vi "AnguloCupula.vi"(2 "ConstantesCupTel":T1={"QtdEtiq"=720, "EtiqMin"=1, "EtiqMax"=720, "Offset"=148.0, "SegurancaAjuste"=2.0, "LargTrapeira"=30.0, "ProjecaoTubo"=20.0, "RaioCupula"=7.525, "DistEntreEixos"=1.57, "AltBase"=0.3, "LATrad"=-0.3933}, 3 "AplicarAjuste":bool=TRUE, 4 "DEC":dbl, 5 "AH":dbl) -> (0 "PosCup":u16, 1 "AngCup":dbl)   [LabVIEW 2012]
panel:
  out "Aj_otimo":dbl
  # "(radianos)"
  # "(radianos)"
  # "(num. etiqueta)"
  # "(graus)"
  # "(graus)"
  # "Não"
  # "Sim"
  # "(graus)"
  # "(graus)"
  # "(metros)"
  # "(metros)"
  # "(metros)"
  # "(radianos)"
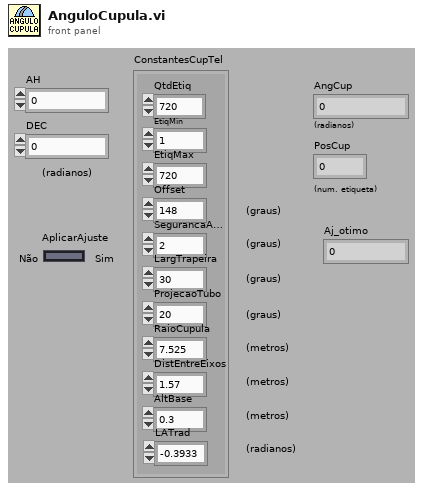
[diagram p1: front panel]
types:
  T1 = cluster{"QtdEtiq":u16, "EtiqMin":u16, "EtiqMax":u16, "Offset":dbl, "SegurancaAjuste":dbl, "LargTrapeira":dbl, "ProjecaoTubo":dbl, "RaioCupula":dbl, "DistEntreEixos":dbl, "AltBase":dbl, "LATrad":dbl}
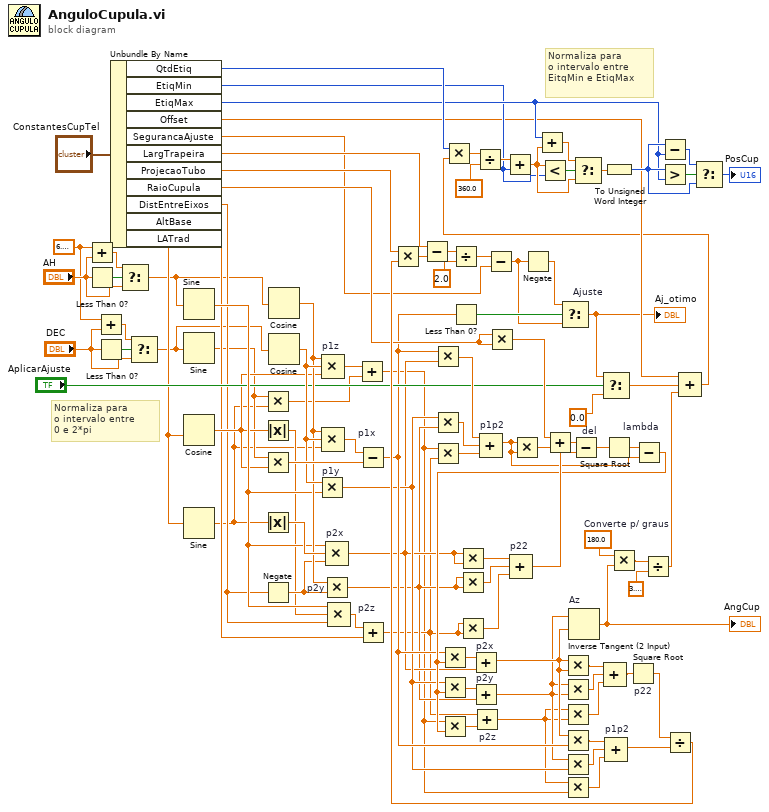
[diagram p0: block diagram]
diagram:
  w2 = 6.283185307179586
  w50 = 180.0  # Converte p/ graus
  # "Normaliza para\no intervalo entre\n0 e 2*pi"
  # "Normaliza para\no intervalo entre\nEitqMin e EtiqMax"
  n1 = Add(x=w2, y="AH") -> (x+y=w6:dbl)
  n2 = Less Than 0?(x="AH") -> (x < 0?=w9:bool)
  n3 = Add(x=w2, y="DEC") -> (x+y=w4:dbl)
  n4 = Less Than 0?(x="DEC") -> (x < 0?=w5:bool)
  n5 = Unbundle By Name("ConstantesCupTel") -> ("QtdEtiq"=w38:u16, "EtiqMin"=w30:u16, "EtiqMax"=w31:u16, "Offset"=w29:dbl, "SegurancaAjuste"=w28:dbl, "LargTrapeira"=w44:dbl, "ProjecaoTubo"=w43:dbl, "RaioCupula"=w42:dbl, "DistEntreEixos"=w41:dbl, "AltBase"=w40:dbl, "LATrad"=w39:dbl)
  n6 = Select(t=w6, s=w9, f="AH") -> (s? t:f=w8:dbl)
  n7 = Select(t=w4, s=w5, f="DEC") -> (s? t:f=w1:dbl)
  n8 = Sine(x=w8) -> (sin(x)=w93:dbl)
  n9 = Sine(x=w1) -> (sin(x)=w12:dbl)
  n10 = Cosine(x=w39) -> (cos(x)=w57:dbl)
  n11 = Sine(x=w39) -> (sin(x)=w11:dbl)
  n12 = Multiply(x=w12, y=w11) -> (x*y=w10:dbl)
  n13 = Absolute Value(x=w57) -> (abs(x)=w13:dbl)
  n14 = Multiply(x=w12, y=w57) -> (x*y=w99:dbl)
  n15 = Absolute Value(x=w11) -> (abs(x)=w95:dbl)
  n16 = Negate(x=w41) -> (-x=w91:dbl)
  n17 = Cosine(x=w8) -> (cos(x)=w94:dbl)
  n18 = Cosine(x=w1) -> (cos(x)=w97:dbl)
  n19 = Multiply "p1y"(x=w97, y=w93) -> (x*y=w25:dbl)
  n20 = Compound Arithmetic op=MULTIPLY "p1z"(w94, w97, w57) -> (w24:dbl)
  n21 = Compound Arithmetic op=MULTIPLY(w94, w97, w11) -> (w98:dbl)
  n22 = Multiply "p2y"(x=w94, y=w91) -> (x*y=w22:dbl)
  n23 = Compound Arithmetic op=MULTIPLY "p2x"(w93, w95, w91) -> (w23:dbl)
  n24 = Compound Arithmetic op=MULTIPLY(w93, w13, w41) -> (w96:dbl)
  n25 = Add(x=w24, y=w10) -> (x+y=w14:dbl)
  n26 = Subtract "p1x"(x=w98, y=w99) -> (x-y=w26:dbl)
  n27 = Add "p2z"(x=w96, y=w40) -> (x+y=w21:dbl)
  n28 = Multiply(x=w26, y=w23) -> (x*y=w86:dbl)
  n29 = Multiply(x=w25, y=w22) -> (x*y=w87:dbl)
  n30 = Multiply(x=w14, y=w21) -> (x*y=w92:dbl)
  n31 = Less Than 0?(x=w26) -> (x < 0?=w66:bool)
  n32 = Multiply(x=w23, y=w23) -> (x*y=w90:dbl)
  n33 = Multiply(x=w22, y=w22) -> (x*y=w89:dbl)
  n34 = Multiply(x=w21, y=w21) -> (x*y=w88:dbl)
  n35 = Compound Arithmetic op=ADD "p1p2"(w86, w87, w92) -> (w79:dbl)
  n36 = Multiply(x=w42, y=w42) -> (x*y=w83:dbl)
  n37 = Compound Arithmetic op=ADD "p22"(w90, w89, w88) -> (w82:dbl)
  n38 = Multiply(x=w79, y=w79) -> (x*y=w85:dbl)
  n39 = Add(x=w83, y=w85) -> (x+y=w84:dbl)
  n40 = Subtract "del"(x=w84, y=w82) -> (x-y=w81:dbl)
  n41 = Square Root(x=w81) -> (sqrt(x)=w80:dbl)
  n42 = Subtract "lambda"(x=w80, y=w79) -> (x-y=w60:dbl)
  n43 = Multiply(x=w26, y=w60) -> (x*y=w61:dbl)
  n44 = Multiply(x=w25, y=w60) -> (x*y=w78:dbl)
  n45 = Multiply(x=w14, y=w60) -> (x*y=w62:dbl)
  n46 = Add "p2x"(x=w61, y=w23) -> (x+y=w20:dbl)
  n47 = Add "p2y"(x=w78, y=w22) -> (x+y=w19:dbl)
  n48 = Add "p2z"(x=w21, y=w62) -> (x+y=w18:dbl)
  n49 = Multiply(x=w20, y=w20) -> (x*y=w74:dbl)
  n50 = Multiply(x=w19, y=w19) -> (x*y=w72:dbl)
  n51 = Multiply(x=w18, y=w18) -> (x*y=w73:dbl)
  n52 = Multiply(x=w20, y=w26) -> (x*y=w77:dbl)
  n53 = Multiply(x=w19, y=w25) -> (x*y=w75:dbl)
  n54 = Multiply(x=w18, y=w14) -> (x*y=w76:dbl)
  n55 = Inverse Tangent (2 Input) "Az"(1:w20, 2:w19) -> (0:w51:dbl)
  "AngCup" <- w51
  n56 = Compound Arithmetic op=ADD ("p1p2")(w74, w72, w73) -> (w71:dbl)
  n57 = Compound Arithmetic op=ADD "p1p2"(w77, w75, w76) -> (w16:dbl)
  n58 = Multiply(x=w50, y=w51) -> (x*y=w49:dbl)
  n59 = Square Root "p22"(x=w71) -> (sqrt(x)=w17:dbl)
  n60 = Divide(x=w49, y=3.141592653589793) -> (x/y=w47:dbl)
  n61 = Divide(x=w17, y=w16) -> (x/y=w63:dbl)
  n62 = Multiply(x=w43, y=w63) -> (x*y=w70:dbl)
  n63 = Subtract(x=w44, y=w70) -> (x-y=w69:dbl)
  n64 = Divide(x=w69, y=2.0) -> (x/y=w67:dbl)
  n65 = Subtract(x=w67, y=w28) -> (x-y=w64:dbl)
  n66 = Negate(x=w64) -> (-x=w65:dbl)
  n67 = Select "Ajuste"(t=w65, s=w66, f=w64) -> (s? t:f=w15:dbl)
  "Aj_otimo" <- w15
  n68 = Select(t=w15, s="AplicarAjuste", f=0.0) -> (s? t:f=w46:dbl)
  n69 = Compound Arithmetic op=ADD(w29, w46, w47) -> (w27:dbl)
  n70 = Multiply(x=w38, y=w27) -> (x*y=w37:dbl)
  n71 = Divide(x=w37, y=360.0) -> (x/y=w34:dbl)
  n72 = Add(x=w34, y=w30) -> (x+y=w35:dbl)
  n73 = Add(x=w31, y=w35) -> (x+y=w56:dbl)
  n74 = Less?(x=w35, y=w30) -> (x < y?=w52:bool)
  n75 = Select(t=w56, s=w52, f=w35) -> (s? t:f=w33:dbl)
  n76 = To Unsigned Word Integer(number=w33) -> (unsigned 16bit integer=w32:u16)
  n77 = Subtract(x=w32, y=w31) -> (x-y=w54:u16)
  n78 = Greater?(x=w32, y=w31) -> (0:w55:bool)
  n79 = Select(t=w54, s=w55, f=w32) -> (s? t:f=→"PosCup":u16)
